vi "Close.vi"(8 "error in":errorcluster, 11 "Cycler in":refnum<class "Cycler.lvclass">) -> (0 "error out":errorcluster, 3 "Cycler out":refnum<class "Cycler.lvclass">)   [LabVIEW 2023, in "Cycler.lvclass"]
uses:
  Cycler.lvclass
  Cycler.lvclass/Cycler.ctl
  <vilib>/ADAS Replay HIL/AdasHilServices/AdasHilServices Fill In Error Info Ex.vi
  <vilib>/ADAS Replay HIL/AdasHilServices/AdasHilChannelServices.lvlib
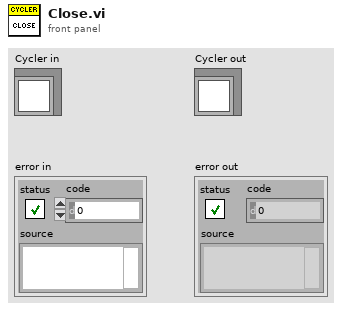
[diagram p1: front panel]
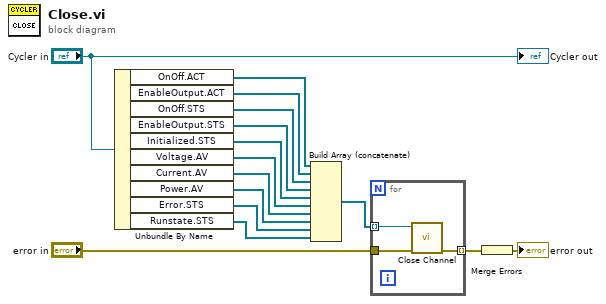
[diagram p0: block diagram]
diagram:
  n1 = Unbundle By Name("Cycler in") -> ("OnOff.ACT"=w11:refnum<k21>[], "EnableOutput.ACT"=w10:refnum<k21>[], "OnOff.STS"=w9:refnum<k21>[], "EnableOutput.STS"=w8:refnum<k21>[], "Initialized.STS"=w7:refnum<k21>[], "Voltage.AV"=w6:refnum<k21>[], "Current.AV"=w5:refnum<k21>[], "Power.AV"=w4:refnum<k21>[], "Error.STS"=w2:refnum<k21>[], "Runstate.STS"=w1:refnum<k21>[])
  n2 = Build Array (concatenate)(w11, w10, w9, w8, w7, w6, w5, w4, w2, w1) -> (w3:refnum<k21>[])
  n3 = for {
    tunnel: w3 -> [w16] mode=indexing
    tunnel: "error in" -> [w18]
    tunnel: [w17] -> w13 mode=indexing
    n4 = call <vilib>:"Close Channel.vi"("error in"=w18, "ADAS HIL Channel"=w16) -> ("error out"=w17:errorcluster)  [unwired: 9 in]
  }
  n5 = Merge Errors(w13) -> (→"error out":errorcluster)
  "Cycler out" <- "Cycler in"
